vi "testTestCaseExecuted.vi"(8 "error in (no error)":errorcluster) -> (0 "error out":errorcluster)   [LabVIEW 2019, in "TestSuiteTest.lvlib" / "Run.lvlib"]
uses:
  Run.lvlib
  TestSuite/TestSuite.lvclass
  TestSuiteTestSupport/TestCaseMock/TestCaseMock.lvclass
  TestResult/TestResult.lvclass
  Assertion/Assertion.lvlib
  C:/Users/de200256/Code/LVUnit/TestCase/TestCase/TestCase.lvclass
  TestCase/TestCase/TestCase.lvclass
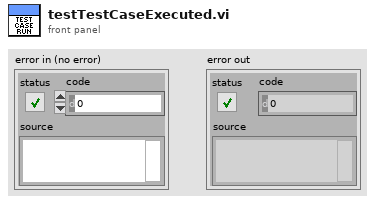
[diagram p1: front panel]
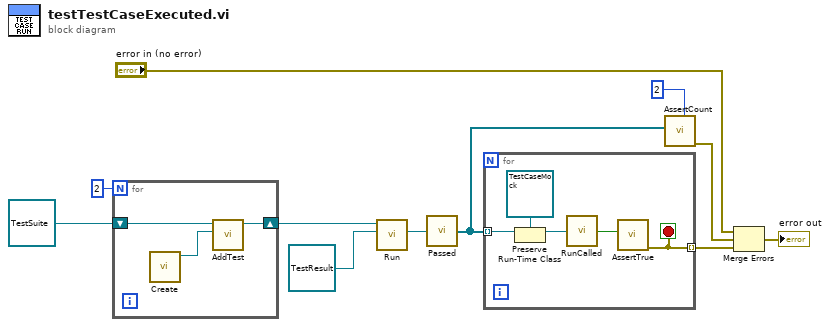
[diagram p0: block diagram]
diagram:
  n1 = for {
    N: 2 -> [_]
    shift-right: [w13] -> w8
    shift-left: refnum<class "TestSuite.lvclass"> refnum ("TestSuite.lvclass") -> [w14]
    n2 = call "Create.vi"() -> ("TestCaseMock"=w12:refnum<class "TestCaseMock.lvclass">)  [unwired: 10 in, 1 out]
    n3 = call-dynamic "AddTest.vi"("TestCase"=w12, "TestSuite in"=w14) -> ("TestSuite out"=w13:refnum<class "TestSuite.lvclass">)  [unwired: 8 in, 1 out]
  }
  n4 = call-dynamic "Run.vi"("TestResult"=refnum<class "TestResult.lvclass"> refnum ("TestResult.lvclass"), "TestSuite in"=w8) -> ("TestResult out"=w6:refnum<class "TestResult.lvclass">)  [unwired: 7 in, 2 out]
  n5 = call "Passed.vi"("TestResult In"=w6) -> ("Passed"=w2:refnum<class "TestCase.lvclass">[])
  n6 = for {
    tunnel: w2 -> [w19] mode=indexing
    tunnel: [w15] -> w5 mode=indexing
    stop <- w15 stop-if-true
    n7 = Preserve Run-Time Class(object in=w19, 2:refnum<class "TestCaseMock.lvclass"> refnum ("TestCaseMock")) -> (object out=w17:refnum<class "TestCaseMock.lvclass">)  [unwired: 1 in, 1 out]
    n8 = call "RunCalled.vi"("TestCaseMock In"=w17) -> ("Run Called"=w16:bool)
    n9 = call "AssertTrue.vi"("Condition"=w16) -> ("error out"=w15:errorcluster)  [unwired: 10 in]
  }
  n10 = call "AssertCount.vi"("Expected"=2, "Haystack"=w2) -> ("error out"=w3:errorcluster)  [unwired: 9 in]
  n11 = Merge Errors("error in (no error)", w3, w5) -> (→"error out":errorcluster)
